vi "CTRE_PigeonIMU_Global.vi"(6 "Set Boolean":bool, 7 "Write After Receive":T2={"PigeonState"=enum."NoComm", "FusedHeading"={"Heading"=0.0, "Valid?"=TRUE, "Fusing?"=TRUE}, "YPR"={"Yaw"=0.0, "Pitch"=0.0, "Roll"=0.0}, "Compass"={"Heading"=0.0, "Magnitude"=0.0, "Absolute Heading"=0.0}, "Accelerometer"={"Biased"={"X"=0, "Y"=0, "Z"=0, "Norm"=0}, "Angles"={"XZ Tilt"=0.0, "YZ Tilt"=0.0, "XY Tilt"=0.0}}, "Magnetometer"={"Raw"={"X"=0, "Y"=0, "Z"=0}, "Biased"={"X"=0, "Y"=0, "Z"=0}}, "Gyro"={"X"=0.0, "Y"=0.0, "Z"=0.0, "Norm"=0.0}, "6D Quaternian"={"W"=0.0, "X"=0.0, "Y"=0.0, "Z"=0.0}, "Temp. (C)"=0.0, "UpTime"=0, "StartupStatus"={"ResetCount"=0, "ResetFlags"=0, "FirmwareVersion"=0, "HasReset?"=TRUE}, "Calibration"={"CurrentMode"=0, "LastCalError"=0, "CalBooting?"=TRUE}, "CAN Error"={"status"=FALSE, "code"=0, "source"=""}, "AccumGyro"={"X"=0.0, "Y"=0.0, "Z"=0.0}} {"Calibration"."CurrentMode" items=["BootTareGryoAccel"=0, "Temperature"=1, "Magnetometer12Pt"=2, "Magnetometer360"=3, "Accelerometer"=5]}, 8 "Set Number":dbl, 10 "Operation":T1, 11 "Device ID (0)":u8) -> (1 "Get All":T2={"PigeonState"=enum."NoComm", "FusedHeading"={"Heading"=0.0, "Valid?"=TRUE, "Fusing?"=TRUE}, "YPR"={"Yaw"=0.0, "Pitch"=0.0, "Roll"=0.0}, "Compass"={"Heading"=0.0, "Magnitude"=0.0, "Absolute Heading"=0.0}, "Accelerometer"={"Biased"={"X"=0, "Y"=0, "Z"=0, "Norm"=0}, "Angles"={"XZ Tilt"=0.0, "YZ Tilt"=0.0, "XY Tilt"=0.0}}, "Magnetometer"={"Raw"={"X"=0, "Y"=0, "Z"=0}, "Biased"={"X"=0, "Y"=0, "Z"=0}}, "Gyro"={"X"=0.0, "Y"=0.0, "Z"=0.0, "Norm"=0.0}, "6D Quaternian"={"W"=0.0, "X"=0.0, "Y"=0.0, "Z"=0.0}, "Temp. (C)"=0.0, "UpTime"=0, "StartupStatus"={"ResetCount"=0, "ResetFlags"=0, "FirmwareVersion"=0, "HasReset?"=TRUE}, "Calibration"={"CurrentMode"=0, "LastCalError"=0, "CalBooting?"=TRUE}, "CAN Error"={"status"=FALSE, "code"=0, "source"=""}, "AccumGyro"={"X"=0.0, "Y"=0.0, "Z"=0.0}} {"Calibration"."CurrentMode" items=["BootTareGryoAccel"=0, "Temperature"=1, "Magnetometer12Pt"=2, "Magnetometer360"=3, "Accelerometer"=5]}, 3 "Device ID Out":u8, 5 "Read For Send":T5)   [LabVIEW 2016]
uses:
  <vilib>/Rock Robotics/WPI/ThirdParty/Sensors/Pigeon IMU/CTRE_PigeonIMU_GlobalControl.ctl
  <vilib>/Rock Robotics/WPI/ThirdParty/Sensors/Pigeon IMU/CTRE_PigeonIMU_GlobalStatus.ctl
  <vilib>/Rock Robotics/WPI/ThirdParty/Sensors/Pigeon IMU/CTRE_PigeonIMU_PigeonState.ctl
  <vilib>/Rock Robotics/WPI/ThirdParty/Sensors/Pigeon IMU/CTRE_PigeonIMU_CalibrationMode.ctl
  <vilib>/Rock Robotics/WPI/ThirdParty/Sensors/Pigeon IMU/CTRE_PigeonIMU_GlobalOps.ctl
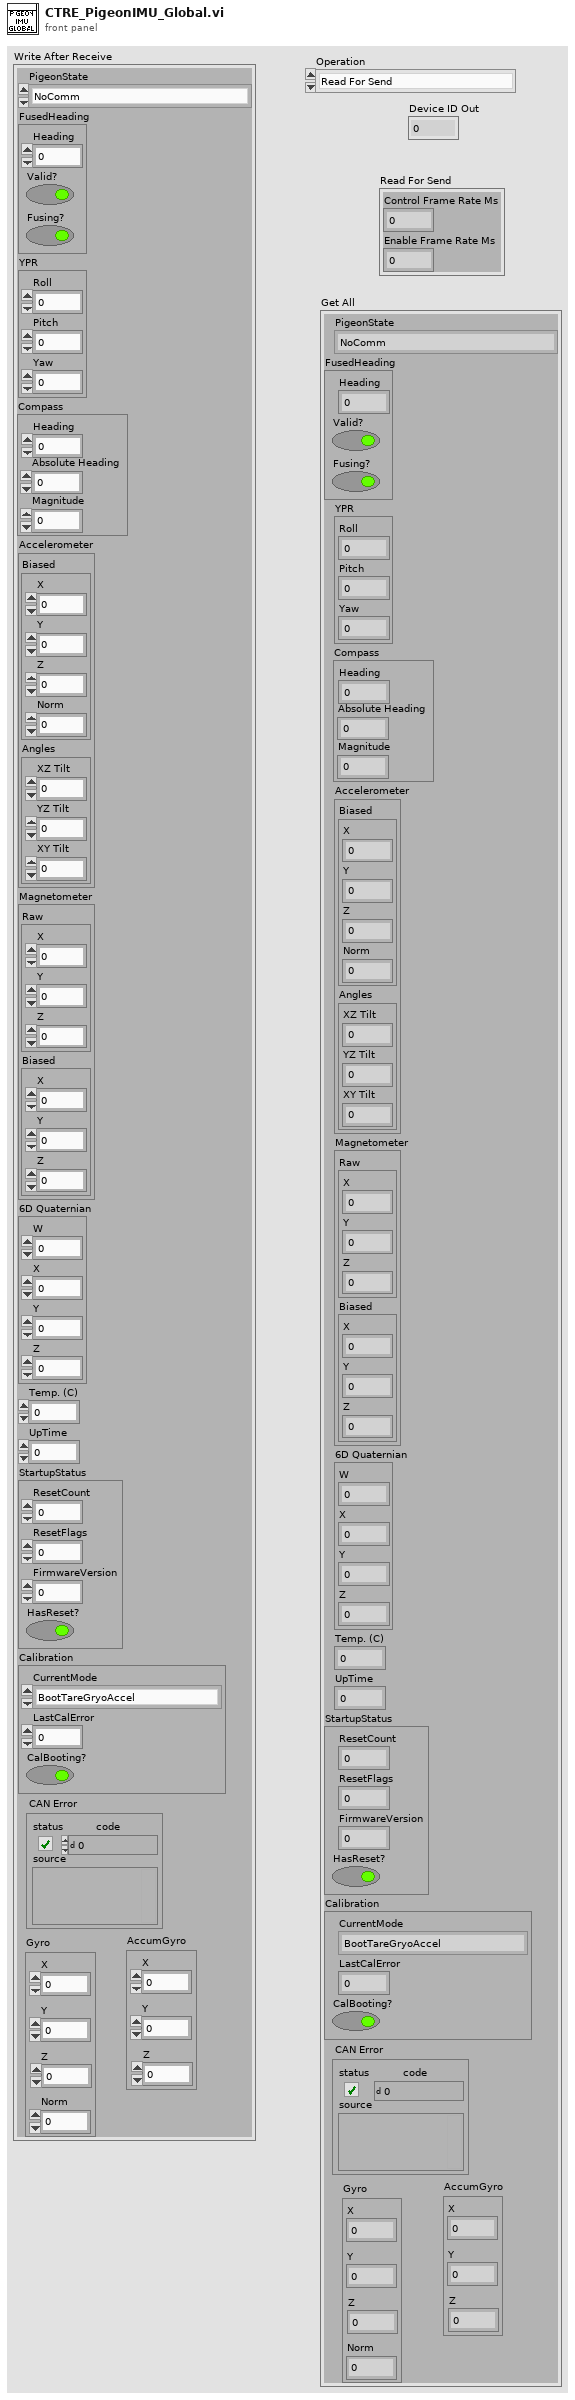
[diagram p1: front panel]
types:
  T1 = typedef "CTRE_PigeonIMU_GlobalOps.ctl" = enum16{"Read For Send", "Write Error", "Get All", "Set Control Frame Rate", "Set Enable Frame Rate", "Write After Receive Fused Heading", "Write After Receive YPR", "Write After Receive Status", "Write After Receive Raw Magnetomoter", "Write After Receive Biased Magnetometer", "Write After Receive Biased Accelerometer", "Write After Receive Gyro", "Write After Receive Acceleromter Angles", "Write After Receive Startup Status", "Write After Receive Compass", "Write After Receive Quaternian", "Write After Receive AccumGyro"}
  T2 = typedef "CTRE_PigeonIMU_GlobalStatus.ctl" = cluster{"PigeonState":T3, "FusedHeading":cluster{"Heading":dbl, "Valid?":bool, "Fusing?":bool}, "YPR":cluster{"Yaw":dbl, "Pitch":dbl, "Roll":dbl}, "Compass":cluster{"Heading":dbl, "Magnitude":dbl, "Absolute Heading":dbl}, "Accelerometer":cluster{"Biased":cluster{"X":i16, "Y":i16, "Z":i16, "Norm":i16}, "Angles":cluster{"XZ Tilt":dbl, "YZ Tilt":dbl, "XY Tilt":dbl}}, "Magnetometer":cluster{"Raw":cluster{"X":i16, "Y":i16, "Z":i16}, "Biased":cluster{"X":i16, "Y":i16, "Z":i16}}, "Gyro":cluster{"X":dbl, "Y":dbl, "Z":dbl, "Norm":dbl}, "6D Quaternian":cluster{"W":dbl, "X":dbl, "Y":dbl, "Z":dbl}, "Temp. (C)":dbl, "UpTime":u32, "StartupStatus":cluster{"ResetCount":i32, "ResetFlags":i32, "FirmwareVersion":i32, "HasReset?":bool}, "Calibration":cluster{"CurrentMode":T4, "LastCalError":i32, "CalBooting?":bool}, "CAN Error":errorcluster, "AccumGyro":cluster{"X":dbl, "Y":dbl, "Z":dbl}}
  T3 = typedef "CTRE_PigeonIMU_PigeonState.ctl" = enum16{"NoComm", "Initializing", "Ready", "UserCalibration"}
  T4 = typedef "CTRE_PigeonIMU_CalibrationMode.ctl" = u16
  T5 = typedef "CTRE_PigeonIMU_GlobalControl.ctl" = cluster{"Control Frame Rate Ms":i32, "Enable Frame Rate Ms":i32}
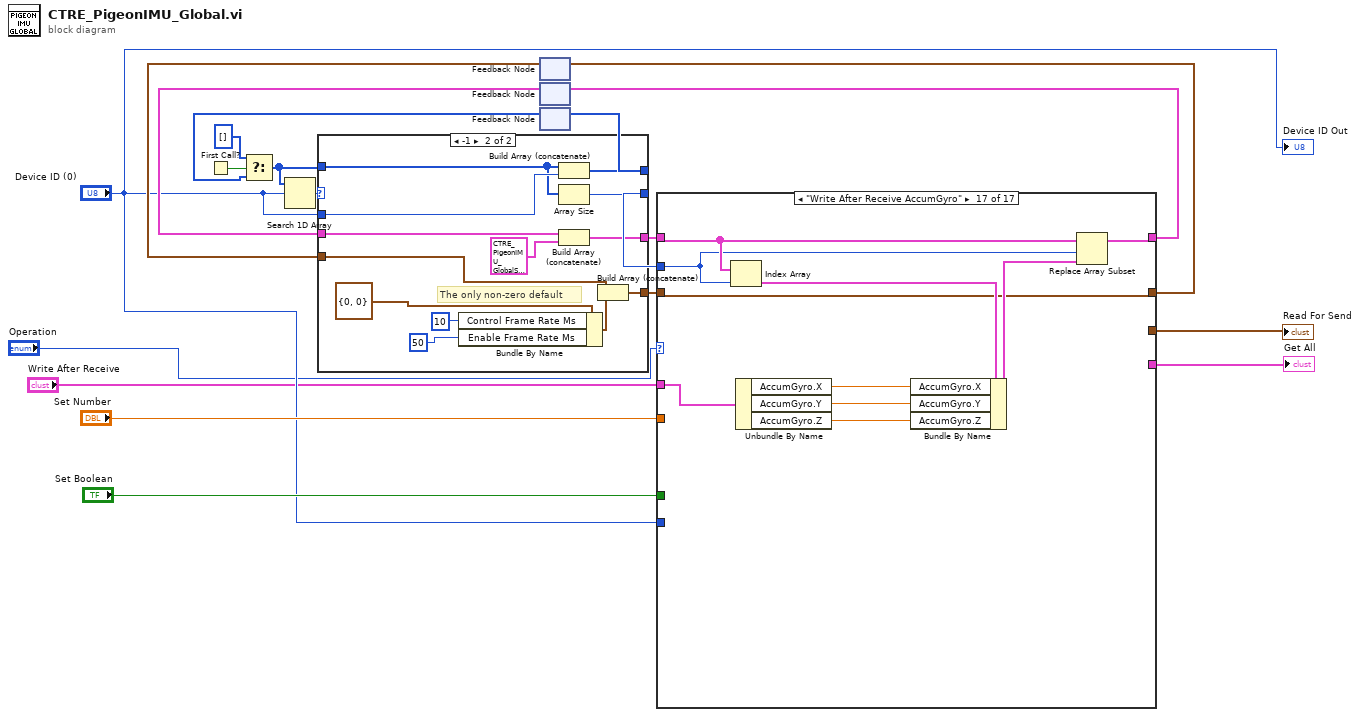
[diagram p0: block diagram]
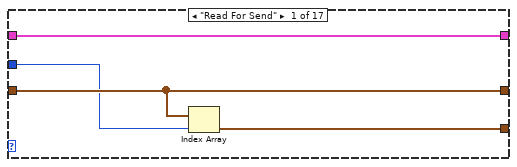
[diagram p2: hidden frame]
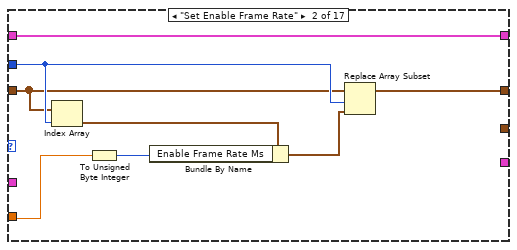
[diagram p3: hidden frame]
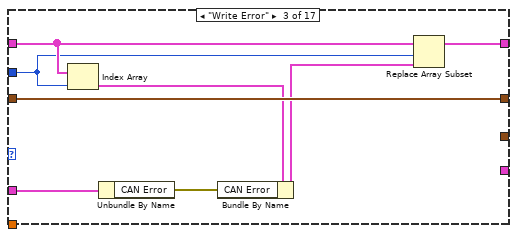
[diagram p4: hidden frame]
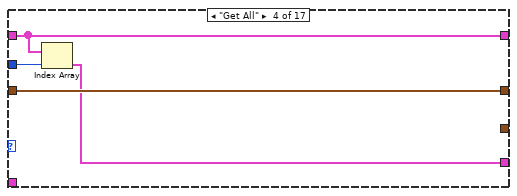
[diagram p5: hidden frame]
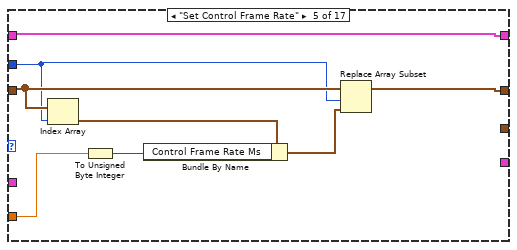
[diagram p6: hidden frame]
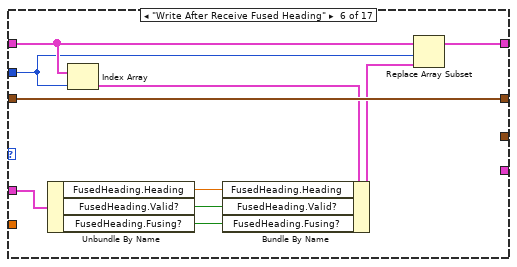
[diagram p7: hidden frame]
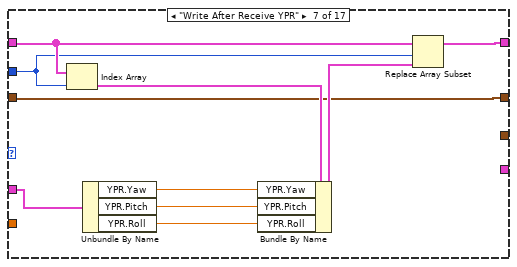
[diagram p8: hidden frame]
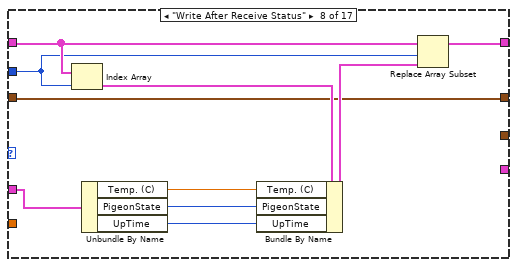
[diagram p9: hidden frame]
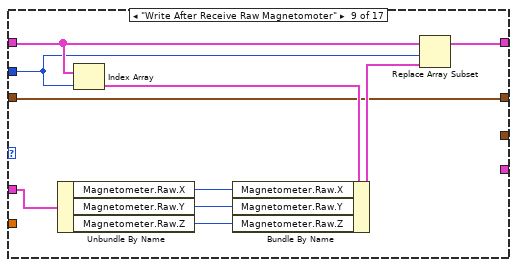
[diagram p10: hidden frame]
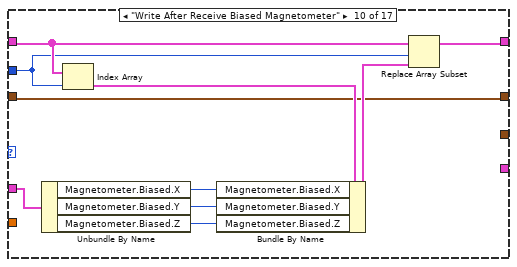
[diagram p11: hidden frame]
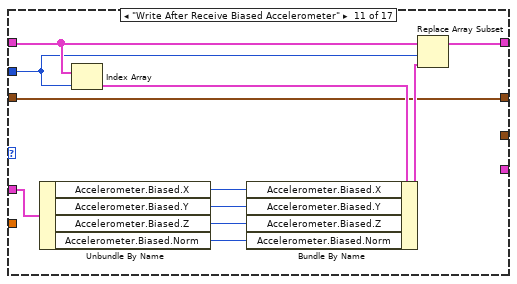
[diagram p12: hidden frame]
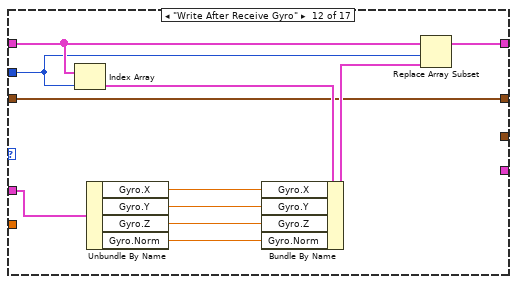
[diagram p13: hidden frame]
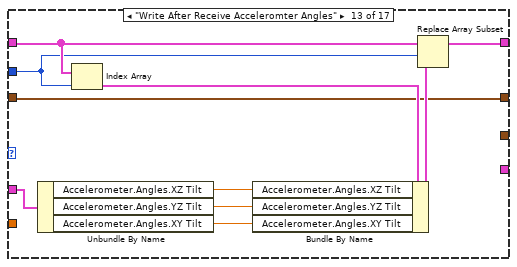
[diagram p14: hidden frame]
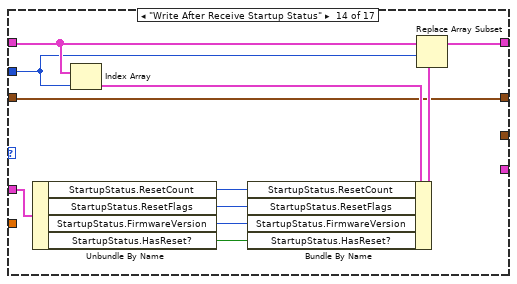
[diagram p15: hidden frame]
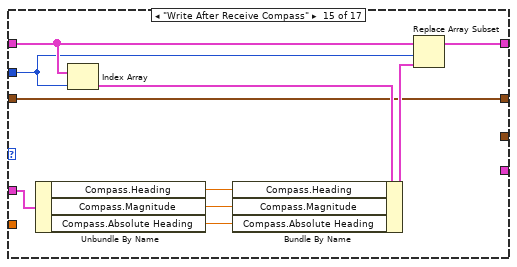
[diagram p16: hidden frame]
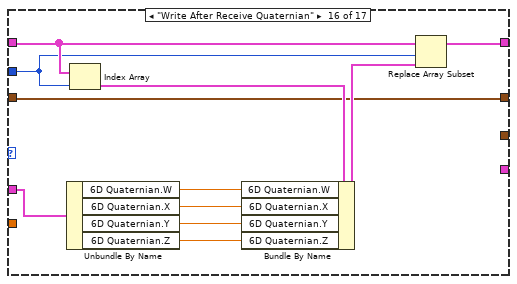
[diagram p17: hidden frame]
diagram:
  n1 = First Call?() -> (First Call?: T/F=w20:bool)
  n2 = feedback #1() -> (w13:T5[])  [unwired: 1 in]
  n3 = feedback #2() -> (w14:T2[])  [unwired: 1 in]
  n4 = feedback #3() -> (w18:u8[])  [unwired: 1 in]
  n5 = Select(t=u8[] [], s=w20, f=w18) -> (s? t:f=w16:u8[])
  n6 = Search 1D Array(1D array=w16, element="Device ID (0)") -> (index of element=w15:i32)  [unwired: 1 in]
  n7 = case shown="-1" w15 {
    selector: w15 -> [w21 _]
    tunnel: [w24 w37] -> w17
    tunnel: "Device ID (0)" -> [_ w36]
    tunnel: w16 -> [w24 w31]
    tunnel: w14 -> [w23 w35]
    tunnel: w13 -> [w22 w34]
    tunnel: [w23 w33] -> w11
    tunnel: [w22 w32] -> w9
    tunnel: [w21 w30] -> w8
    frame Default {
    }
    frame -1 {
      # "The only non-zero default"
      n8 = Bundle By Name(cluster=T5 {"Control Frame Rate Ms"=0, "Enable Frame Rate Ms"=0} ("PigeonIMU Control"), "Control Frame Rate Ms"=u8 10, "Enable Frame Rate Ms"=u8 50) -> (w29:T5)
      n9 = Build Array (concatenate)(w31, w36) -> (w37:u8[])
      n10 = Array Size(array=w31) -> (size(s)=w30:i32)
      n11 = Build Array (concatenate)(w35, T2 {"PigeonState"=enum."NoComm", "FusedHeading"={"Heading"=0.0, "Valid?"=TRUE, "Fusing?"=TRUE}, "YPR"={"Yaw"=0.0, "Pitch"=0.0, "Roll"=0.0}, "Compass"={"Heading"=0.0, "Magnitude"=0.0, "Absolute Heading"=0.0}, "Accelerometer"={"Biased"={"X"=0, "Y"=0, "Z"=0, "Norm"=0}, "Angles"={"XZ Tilt"=0.0, "YZ Tilt"=0.0, "XY Tilt"=0.0}}, "Magnetometer"={"Raw"={"X"=0, "Y"=0, "Z"=0}, "Biased"={"X"=0, "Y"=0, "Z"=0}}, "Gyro"={"X"=0.0, "Y"=0.0, "Z"=0.0, "Norm"=0.0}, "6D Quaternian"={"W"=0.0, "X"=0.0, "Y"=0.0, "Z"=0.0}, "Temp. (C)"=0.0, "UpTime"=0, "StartupStatus"={"ResetCount"=0, "ResetFlags"=0, "FirmwareVersion"=0, "HasReset?"=TRUE}, "Calibration"={"CurrentMode"=0, "LastCalError"=0, "CalBooting?"=TRUE}, "CAN Error"={"status"=FALSE, "code"=0, "source"=""}, "AccumGyro"={"X"=0.0, "Y"=0.0, "Z"=0.0}} ("PigeonIMU Status")) -> (w33:T2[])
      n12 = Build Array (concatenate)(w34, w29) -> (w32:T5[])
    }
  }
  n13 = feedback-in #3(w17) -> ()
  n14 = case shown="\"Write After Receive AccumGyro\"" "Operation" {
    tunnel: [w41 w43 w56 w59 w65 w78 w83 w93 w103 w113 w124 w135 w145 w156 w167 w178 w187] -> w12
    tunnel: w11 -> [w41 w43 w55 w59 w65 w77 w84 w94 w104 w114 w125 w136 w146 w157 w169 w180 w188]
    tunnel: [w40 w42 w57 w61 w67 w79 w82 w91 w101 w111 w122 w133 w144 w154 w166 w177 w185] -> w10
    tunnel: w9 -> [w40 w44 w57 w61 w68 w79 w82 w91 w101 w111 w122 w133 w144 w154 w166 w177 w185]
    tunnel: w8 -> [w39 w45 w54 w60 w66 w76 w81 w92 w102 w112 w123 w134 w142 w155 w168 w179 w186]
    tunnel: [w38 _ _ _ _ _ _ _ _ _ _ _ _ _ _ _ _] -> w4
    tunnel: "Write After Receive" -> [_ _ w51 _ _ w73 w80 w90 w100 w110 w121 w132 w143 w153 w165 w176 w184]
    tunnel: "Set Number" -> [_ w46 _ _ w63 _ _ _ _ _ _ _ _ _ _ _ _]
    tunnel: [_ _ _ w58 _ _ _ _ _ _ _ _ _ _ _ _ _] -> w3
    tunnel: "Set Boolean" -> [_ _ _ _ _ _ _ _ _ _ _ _ _ _ _ _ _]
    tunnel: "Device ID (0)" -> [_ _ _ _ _ _ _ _ _ _ _ _ _ _ _ _ _]
    frame "Read For Send" {
      n15 = Index Array(array=w40, index=w39) -> (element=w38:T5)
    }
    frame "Set Enable Frame Rate" {
      n16 = Index Array(array=w44, index=w45) -> (element=w48:T5)
      n17 = To Unsigned Byte Integer(number=w46) -> (unsigned 8bit integer=w47:u8)
      n18 = Bundle By Name(cluster=w48, "Enable Frame Rate Ms"=w47) -> (w49:T5)
      n19 = Replace Array Subset(array=w44, new element=w49, index=w45) -> (w42:T5[])
    }
    frame "Write Error" {
      n20 = Index Array(array=w55, index=w54) -> (element=w53:T2)
      n21 = Unbundle By Name(w51) -> ("CAN Error"=w50:errorcluster)
      n22 = Bundle By Name(cluster=w53, "CAN Error"=w50) -> (w52:T2)
      n23 = Replace Array Subset(array=w55, new element=w52, index=w54) -> (w56:T2[])
    }
    frame "Get All" {
      n24 = Index Array(array=w59, index=w60) -> (element=w58:T2)
    }
    frame "Set Control Frame Rate" {
      n25 = Index Array(array=w68, index=w66) -> (element=w64:T5)
      n26 = To Unsigned Byte Integer(number=w63) -> (unsigned 8bit integer=w62:u8)
      n27 = Bundle By Name(cluster=w64, "Control Frame Rate Ms"=w62) -> (w69:T5)
      n28 = Replace Array Subset(array=w68, new element=w69, index=w66) -> (w67:T5[])
    }
    frame "Write After Receive Fused Heading" {
      n29 = Unbundle By Name(w73) -> ("FusedHeading.Heading"=w72:dbl, "FusedHeading.Valid?"=w71:bool, "FusedHeading.Fusing?"=w70:bool)
      n30 = Index Array(array=w77, index=w76) -> (element=w75:T2)
      n31 = Bundle By Name(cluster=w75, "FusedHeading.Heading"=w72, "FusedHeading.Valid?"=w71, "FusedHeading.Fusing?"=w70) -> (w74:T2)
      n32 = Replace Array Subset(array=w77, new element=w74, index=w76) -> (w78:T2[])
    }
    frame "Write After Receive YPR" {
      n33 = Index Array(array=w84, index=w81) -> (element=w85:T2)
      n34 = Unbundle By Name(w80) -> ("YPR.Yaw"=w87:dbl, "YPR.Pitch"=w88:dbl, "YPR.Roll"=w89:dbl)
      n35 = Bundle By Name(cluster=w85, "YPR.Yaw"=w87, "YPR.Pitch"=w88, "YPR.Roll"=w89) -> (w86:T2)
      n36 = Replace Array Subset(array=w84, new element=w86, index=w81) -> (w83:T2[])
    }
    frame "Write After Receive Status" {
      n37 = Index Array(array=w94, index=w92) -> (element=w99:T2)
      n38 = Unbundle By Name(w90) -> ("Temp. (C)"=w97:dbl, "PigeonState"=w96:T3, "UpTime"=w95:u32)
      n39 = Bundle By Name(cluster=w99, "Temp. (C)"=w97, "PigeonState"=w96, "UpTime"=w95) -> (w98:T2)
      n40 = Replace Array Subset(array=w94, new element=w98, index=w92) -> (w93:T2[])
    }
    frame "Write After Receive Raw Magnetomoter" {
      n41 = Unbundle By Name(w100) -> ("Magnetometer.Raw.X"=w107:i16, "Magnetometer.Raw.Y"=w106:i16, "Magnetometer.Raw.Z"=w105:i16)
      n42 = Index Array(array=w104, index=w102) -> (element=w109:T2)
      n43 = Bundle By Name(cluster=w109, "Magnetometer.Raw.X"=w107, "Magnetometer.Raw.Y"=w106, "Magnetometer.Raw.Z"=w105) -> (w108:T2)
      n44 = Replace Array Subset(array=w104, new element=w108, index=w102) -> (w103:T2[])
    }
    frame "Write After Receive Biased Magnetometer" {
      n45 = Unbundle By Name(w110) -> ("Magnetometer.Biased.X"=w117:i16, "Magnetometer.Biased.Y"=w116:i16, "Magnetometer.Biased.Z"=w115:i16)
      n46 = Index Array(array=w114, index=w112) -> (element=w119:T2)
      n47 = Bundle By Name(cluster=w119, "Magnetometer.Biased.X"=w117, "Magnetometer.Biased.Y"=w116, "Magnetometer.Biased.Z"=w115) -> (w118:T2)
      n48 = Replace Array Subset(array=w114, new element=w118, index=w112) -> (w113:T2[])
    }
    frame "Write After Receive Biased Accelerometer" {
      n49 = Unbundle By Name(w121) -> ("Accelerometer.Biased.X"=w128:i16, "Accelerometer.Biased.Y"=w127:i16, "Accelerometer.Biased.Z"=w126:i16, "Accelerometer.Biased.Norm"=w120:i16)
      n50 = Index Array(array=w125, index=w123) -> (element=w130:T2)
      n51 = Bundle By Name(cluster=w130, "Accelerometer.Biased.X"=w128, "Accelerometer.Biased.Y"=w127, "Accelerometer.Biased.Z"=w126, "Accelerometer.Biased.Norm"=w120) -> (w129:T2)
      n52 = Replace Array Subset(array=w125, new element=w129, index=w123) -> (w124:T2[])
    }
    frame "Write After Receive Gyro" {
      n53 = Index Array(array=w136, index=w134) -> (element=w141:T2)
      n54 = Unbundle By Name(w132) -> ("Gyro.X"=w139:dbl, "Gyro.Y"=w138:dbl, "Gyro.Z"=w137:dbl, "Gyro.Norm"=w131:dbl)
      n55 = Bundle By Name(cluster=w141, "Gyro.X"=w139, "Gyro.Y"=w138, "Gyro.Z"=w137, "Gyro.Norm"=w131) -> (w140:T2)
      n56 = Replace Array Subset(array=w136, new element=w140, index=w134) -> (w135:T2[])
    }
    frame "Write After Receive Acceleromter Angles" {
      n57 = Unbundle By Name(w143) -> ("Accelerometer.Angles.XZ Tilt"=w149:dbl, "Accelerometer.Angles.YZ Tilt"=w150:dbl, "Accelerometer.Angles.XY Tilt"=w151:dbl)
      n58 = Index Array(array=w146, index=w142) -> (element=w147:T2)
      n59 = Bundle By Name(cluster=w147, "Accelerometer.Angles.XZ Tilt"=w149, "Accelerometer.Angles.YZ Tilt"=w150, "Accelerometer.Angles.XY Tilt"=w151) -> (w148:T2)
      n60 = Replace Array Subset(array=w146, new element=w148, index=w142) -> (w145:T2[])
    }
    frame "Write After Receive Startup Status" {
      n61 = Unbundle By Name(w153) -> ("StartupStatus.ResetCount"=w160:i32, "StartupStatus.ResetFlags"=w159:i32, "StartupStatus.FirmwareVersion"=w158:i32, "StartupStatus.HasReset?"=w152:bool)
      n62 = Index Array(array=w157, index=w155) -> (element=w162:T2)
      n63 = Bundle By Name(cluster=w162, "StartupStatus.ResetCount"=w160, "StartupStatus.ResetFlags"=w159, "StartupStatus.FirmwareVersion"=w158, "StartupStatus.HasReset?"=w152) -> (w161:T2)
      n64 = Replace Array Subset(array=w157, new element=w161, index=w155) -> (w156:T2[])
    }
    frame "Write After Receive Compass" {
      n65 = Unbundle By Name(w165) -> ("Compass.Heading"=w172:dbl, "Compass.Magnitude"=w164:dbl, "Compass.Absolute Heading"=w163:dbl)
      n66 = Index Array(array=w169, index=w168) -> (element=w170:T2)
      n67 = Bundle By Name(cluster=w170, "Compass.Heading"=w172, "Compass.Magnitude"=w164, "Compass.Absolute Heading"=w163) -> (w171:T2)
      n68 = Replace Array Subset(array=w169, new element=w171, index=w168) -> (w167:T2[])
    }
    frame "Write After Receive Quaternian" {
      n69 = Unbundle By Name(w176) -> ("6D Quaternian.W"=w181:dbl, "6D Quaternian.X"=w175:dbl, "6D Quaternian.Y"=w174:dbl, "6D Quaternian.Z"=w173:dbl)
      n70 = Index Array(array=w180, index=w179) -> (element=w183:T2)
      n71 = Bundle By Name(cluster=w183, "6D Quaternian.W"=w181, "6D Quaternian.X"=w175, "6D Quaternian.Y"=w174, "6D Quaternian.Z"=w173) -> (w182:T2)
      n72 = Replace Array Subset(array=w180, new element=w182, index=w179) -> (w178:T2[])
    }
    frame "Write After Receive AccumGyro" {
      n73 = Index Array(array=w188, index=w186) -> (element=w189:T2)
      n74 = Unbundle By Name(w184) -> ("AccumGyro.X"=w191:dbl, "AccumGyro.Y"=w192:dbl, "AccumGyro.Z"=w193:dbl)
      n75 = Bundle By Name(cluster=w189, "AccumGyro.X"=w191, "AccumGyro.Y"=w192, "AccumGyro.Z"=w193) -> (w190:T2)
      n76 = Replace Array Subset(array=w188, new element=w190, index=w186) -> (w187:T2[])
    }
  }
  "Read For Send" <- w4
  "Get All" <- w3
  n77 = feedback-in #1(w10) -> ()
  n78 = feedback-in #2(w12) -> ()
  "Device ID Out" <- "Device ID (0)"
